vi "WAPIAerScopeCommand.vi"(3 "data":u16, 7 "cmd":T1(ring), 9 "error in (no error)":errorcluster) -> (0 "count":i32, 6 "error out":errorcluster)   [LabVIEW 2009]
uses:
  win50032.dll
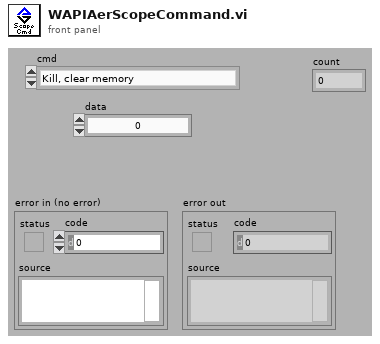
[diagram p1: front panel]
types:
  T1 = enum8{"Kill, clear memory", "Feedback Actual velocity data", "Feedback Command velocity data", "Feedback Auxiliary data", "Set time base (ms)", "Enable Tracking", "Stop Tracking, but keep data", "Set # of samples [1-2500]", "Set auxiliary sample type", "Feedback Auto tune Velocity", "Feedback Auto tune Torque"}
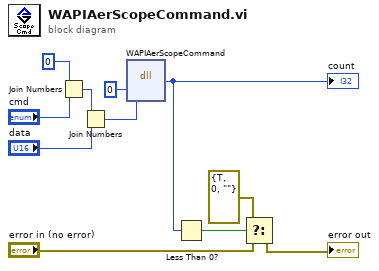
[diagram p0: block diagram]
diagram:
  n1 = Join Numbers(hi=u8 0, lo="cmd") -> ((hi.lo)=w3:u16)
  n2 = Join Numbers(hi=w3, lo="data") -> ((hi.lo)=w2:u32)
  n3 = dll-call lib="Win50032.dll" fn="WAPIAerScopeCommand"("timeout"=0, "cmd"=w2) -> ("return type"=w10:i32)  [unwired: 5 in, 2 out]
  "count" <- w10
  n4 = Less Than 0?(x=w10) -> (x < 0?=w6:bool)
  n5 = Select(t=errorcluster {"status"=TRUE, "code"=0, "source"=""} ("error in (no error)"), s=w6, f="error in (no error)") -> (s? t:f=→"error out":errorcluster)
